vi "Phasor Explorer f(tau) [SEPL Intersections].vi"(4 "data":variant, 5 "x":dbl) -> (2 "f(x)":dbl)   [LabVIEW 2021, in "Phasor Explorer.lvlib"]
uses:
  Phasor Explorer.lvlib
  Phasor.lvlib
  Phasor Gate Definitions.ctl
  Phasor Decay Definiton.ctl
  Phasor Data for SEPL Intersections.ctl
  Phasor Calculation Type.ctl
  Phasor Gate Type.ctl
  Phasor IRF Model.ctl
  Graphs/XY Graph/XY Plot Data.ctl
  Graphs/XY Graph/XY Graph Add-Ons.lvlib
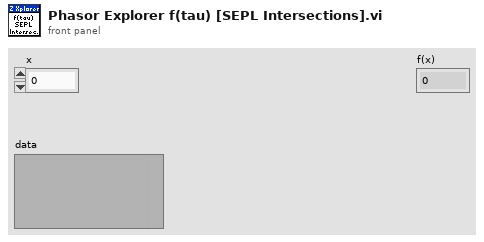
[diagram p1: front panel]
types:
  T1 = typedef "Phasor.lvlib/Phasor Data for SEPL Intersections.ctl" = cluster{"Linear Coefficients":cluster{"u":dbl, "v":dbl}, "Decay Definition":T2, "Gates Definitions":T4, "iw":cdb, "Phasor Calculation":T7}
  T2 = typedef "Phasor.lvlib/Phasor Decay Definiton.ctl" = cluster{"offset: t0":ext, "period: T":ext, "lifetime: tau":ext, "Incident Signal: I":ext, "Normalized Decays":bool, "IRF Model":T3, "IRF Parameter 1":ext, "Poisson Signal":bool}
  T3 = typedef "Phasor.lvlib/Phasor IRF Model.ctl" = enum16{"Dirac", "Exponential"}
  T4 = typedef "Phasor.lvlib/Phasor Gate Definitions.ctl" = cluster{"First Gate: t1":ext, "Gate Width: W":ext, "Gate Step: d":ext, "# Gates: G":ext, "Use Gate Center":bool, "Frames/Image: F":i32, "Gates/Frame: L":i32, "Bits/Frame: q":i32, "Multiplicity: p":i32, "Gate Type":T5, "Gate Edge s":ext, "Gate Top Slope":ext, "Reversed Sawtooth?":bool, "Computation":bool, "User-defined Gate":T6, "Tolerance":ext, "Integration":enum32{"Item 0", "Item 1"}, "# Steps":ext, "Type of User-defined Function":enum32{"Gate", "IRF"}}
  T5 = typedef "Phasor.lvlib/Phasor Gate Type.ctl" = enum16{"Square", "Finite Edge Square", "Finite Edge, Tilted Top Square", "Triangle", "Sawtooth", "User-defined"}
  T6 = typedef "XY Graph Add-Ons.lvlib/XY Plot Data.ctl" = cluster{"X Array":dbl[], "Y Array":dbl[]}
  T7 = typedef "Phasor.lvlib/Phasor Calculation Type.ctl" = enum16{"Direct Sum", "Analytical Formula"}
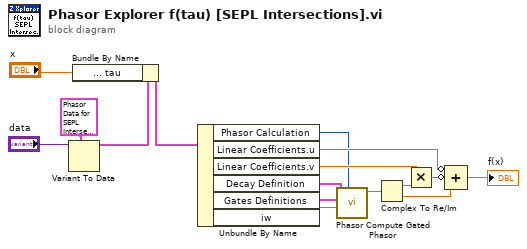
[diagram p0: block diagram]
diagram:
  n1 = Variant To Data(type=T1 {"Linear Coefficients"={"u"=0.0, "v"=0.0}, "Decay Definition"={"offset: t0"=0.0, "period: T"=0.0, "lifetime: tau"=0.0, "Incident Signal: I"=0.5, "Normalized Decays"=FALSE, "IRF Model"=enum."Dirac", "IRF Parameter 1"=0.0, "Poisson Signal"=FALSE}, "Gates Definitions"={"First Gate: t1"=0.0, "Gate Width: W"=0.0, "Gate Step: d"=0.0, "# Gates: G"=0.0, "Use Gate Center"=FALSE, "Frames/Image: F"=50, "Gates/Frame: L"=0, "Bits/Frame: q"=0, "Multiplicity: p"=0, "Gate Type"=enum."Square", "Gate Edge s"=4.0, "Gate Top Slope"=4.0, "Reversed Sawtooth?"=FALSE, "Computation"=FALSE, "User-defined Gate"={"X Array"=[], "Y Array"=[]}, "Tolerance"=50.0, "Integration"=enum."Item 0", "# Steps"=50.0, "Type of User-defined Function"=enum."Gate"}, "iw"=0.0+0.0i, "Phasor Calculation"=enum."Direct Sum"} ("cluster"), Variant="data") -> (data=w4:T1)  [unwired: 1 in, 1 out]
  n2 = Bundle By Name(cluster=w4, "Decay Definition.lifetime: tau"="x") -> (w7:T1)
  n3 = Unbundle By Name(w7) -> ("Phasor Calculation"=w1:T7, "Linear Coefficients.u"=w11:dbl, "Linear Coefficients.v"=w12:dbl, "Decay Definition"=w10:T2, "Gates Definitions"=w9:T4, "iw"=w8:cdb)
  n4 = call "Phasor Compute Gated Phasor.vi"("Phasor Calculation Type"=w1, "j 2 pi f"=w8, "Gates Definitions"=w9, "Decay Definition"=w10) -> ("phasor"=w13:cxt)  [unwired: 5 in, 2 out]
  n5 = Complex To Re/Im(x + iy=w13) -> (x=w16:ext, y=w14:ext)
  n6 = Multiply(x=w12, y=w16) -> (x*y=w15:ext)
  n7 = Compound Arithmetic op=ADD(invert w11, invert w15, w14) -> (→"f(x)":ext)
